vi "int.vi"() -> ()   [LabVIEW 2016]
panel:
  out "数值":i32
  out "元素":i32
  in  "停止":bool
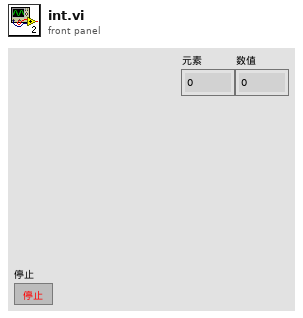
[diagram p1: front panel]
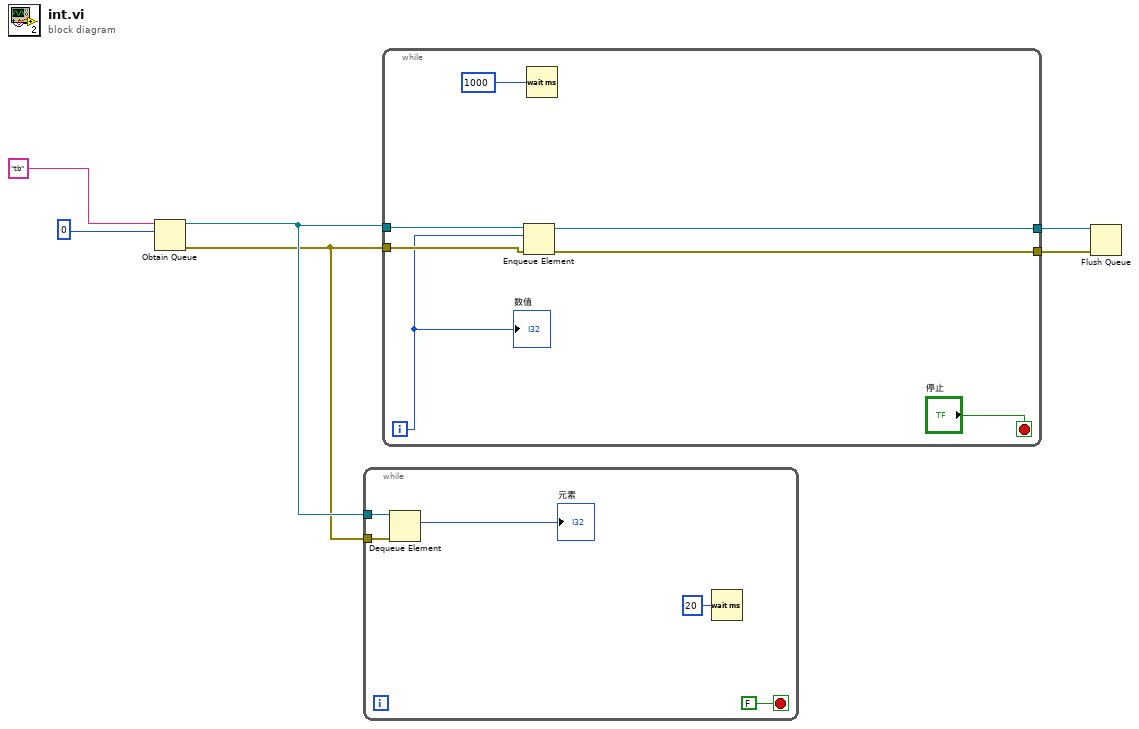
[diagram p0: block diagram]
diagram:
  n1 = Obtain Queue(name (unnamed)="tb" ("名称（未命名）"), element data type=0) -> (queue out=w4:refnum<queue>, error out=w1:errorcluster)  [unwired: 3 in, 1 out]
  n2 = while {
    tunnel: w4 -> [w11]
    tunnel: w1 -> [w10]
    stop <- FALSE stop-if-true
    n3 = Dequeue Element(queue=w11, error in (no error)=w10) -> (element=→"元素":i32)  [unwired: 1 in, 3 out]
    n4 = Wait (ms)(milliseconds to wait=u32 20 ("等待时间（毫秒）")) -> ()  [unwired: 1 out]
  }
  n5 = while {
    tunnel: w4 -> [w16]
    tunnel: w1 -> [w15]
    tunnel: [w14] -> w3
    tunnel: [w13] -> w2
    i -> [w12]
    stop <- "停止" stop-if-true
    n6 = Enqueue Element(queue=w16, element=w12, error in (no error)=w15) -> (queue out=w13:refnum<queue>, error out=w14:errorcluster)  [unwired: 1 in, 1 out]
    n7 = Wait (ms)(milliseconds to wait=u32 1000 ("等待时间（毫秒）")) -> ()  [unwired: 1 out]
    "数值" <- w12
  }
  n8 = Flush Queue(queue=w2, error in (no error)=w3) -> ()  [unwired: 3 out]
